vi "Get default digital audio protocol settings.vi"(11 "PCM Interfaces":T6) -> (3 "digital audio protocol settings":T1={"number of channels"=0, "data justification"=enum."Left Justified", "endianness"=enum."LSB First", "channel length"=0, "bit depth"=0, "frame clock rate"=0.0, "bit clock edge sync"=enum."Falling", "master clock rate"=0.0, "Logic Level"=enum."1.2 V", "frame sync edge for channel 0"=enum."Rising", "Channel 0 Offset"=0})   [LabVIEW 2021]
uses:
  Program Files/National Instruments/LabVIEW 2021/examples/Digital Audio Acquisition and Generation Toolkit/subVIs/PCM Interface Type.ctl
  digital audio protocol settings.ctl
  <vilib>/PDM Acquisition Toolkit/shared/controls/PCM Data Justification.ctl
  <vilib>/PDM Acquisition Toolkit/shared/controls/PCM Bit Endianness.ctl
  <vilib>/PDM Acquisition Toolkit/shared/controls/Digital Edge.ctl
  <vilib>/PDM Acquisition Toolkit/host/Classes/Session/Controls/Logic Levels.ctl
  <vilib>/PDM Acquisition Toolkit/shared/PDM Shared.lvlib
  <vilib>/PDM Acquisition Toolkit/host/Classes/Session/DecoderSession.lvclass
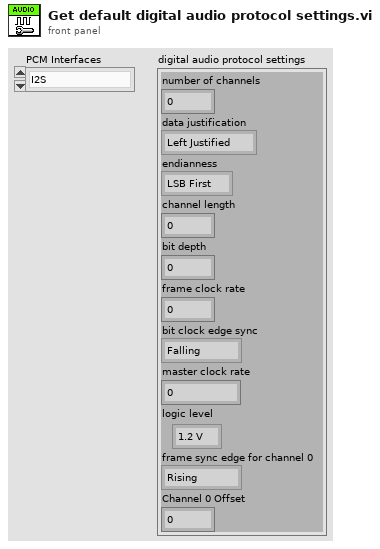
[diagram p1: front panel]
types:
  T1 = typedef "digital audio protocol settings.ctl" = cluster{"number of channels":u16, "data justification":T2, "endianness":T3, "channel length":u16, "bit depth":u8, "frame clock rate":dbl, "bit clock edge sync":T4, "master clock rate":dbl, "Logic Level":T5, "frame sync edge for channel 0":T4, "Channel 0 Offset":u16}
  T2 = typedef "PDM Shared.lvlib/PCM Data Justification.ctl" = enum16{"Left Justified", "Right Justified"}
  T3 = typedef "PDM Shared.lvlib/PCM Bit Endianness.ctl" = enum16{"MSB First", "LSB First"}
  T4 = typedef "PDM Shared.lvlib/Digital Edge.ctl" = enum8{"Rising", "Falling"}
  T5 = typedef "PDM Acquisition Class Library.lvlib/DecoderSession.lvclass/Logic Levels.ctl" = enum16{"3.3 V", "1.8 V", "1.2 V"}
  T6 = typedef "PCM Interface Type.ctl" = enum16{"I2S", "Left Justified", "Right Justified", "TDM 4 Channel", "TDM 6 Channel", "TDM 8 Channel", "DSP mode", "DSP mode with 1 bit delay", "PCM Short Frame", "PCM Long Frame"}
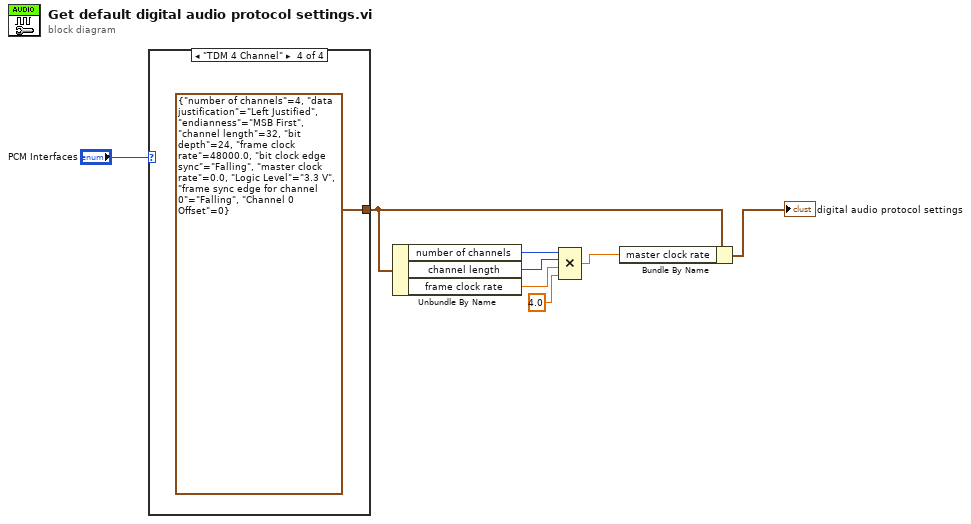
[diagram p0: block diagram]
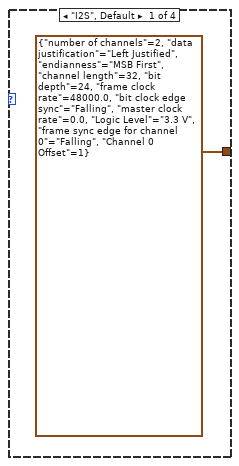
[diagram p2: hidden frame]
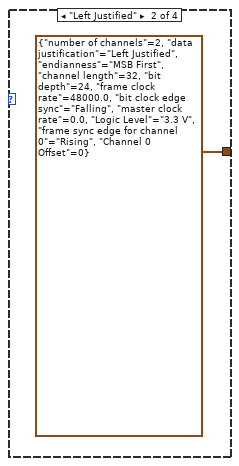
[diagram p3: hidden frame]
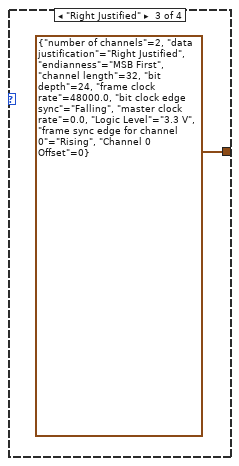
[diagram p4: hidden frame]
diagram:
  n1 = case shown="\"TDM 4 Channel\"" "PCM Interfaces" {
    tunnel: [T1 {"number of channels"=2, "data justification"=enum."Left Justified", "endianness"=enum."MSB First", "channel length"=32, "bit depth"=24, "frame clock rate"=48000.0, "bit clock edge sync"=enum."Falling", "master clock rate"=0.0, "Logic Level"=enum."3.3 V", "frame sync edge for channel 0"=enum."Falling", "Channel 0 Offset"=1} ("Cluster") T1 {"number of channels"=2, "data justification"=enum."Left Justified", "endianness"=enum."MSB First", "channel length"=32, "bit depth"=24, "frame clock rate"=48000.0, "bit clock edge sync"=enum."Falling", "master clock rate"=0.0, "Logic Level"=enum."3.3 V", "frame sync edge for channel 0"=enum."Rising", "Channel 0 Offset"=0} ("Cluster") T1 {"number of channels"=2, "data justification"=enum."Right Justified", "endianness"=enum."MSB First", "channel length"=32, "bit depth"=24, "frame clock rate"=48000.0, "bit clock edge sync"=enum."Falling", "master clock rate"=0.0, "Logic Level"=enum."3.3 V", "frame sync edge for channel 0"=enum."Rising", "Channel 0 Offset"=0} ("Cluster") T1 {"number of channels"=4, "data justification"=enum."Left Justified", "endianness"=enum."MSB First", "channel length"=32, "bit depth"=24, "frame clock rate"=48000.0, "bit clock edge sync"=enum."Falling", "master clock rate"=0.0, "Logic Level"=enum."3.3 V", "frame sync edge for channel 0"=enum."Falling", "Channel 0 Offset"=0} ("Cluster")] -> w7
    frame "I2S", Default {
    }
    frame "Left Justified" {
    }
    frame "Right Justified" {
    }
    frame "TDM 4 Channel" {
    }
  }
  n2 = Unbundle By Name(w7) -> ("number of channels"=w5:u16, "channel length"=w4:u16, "frame clock rate"=w3:dbl)
  n3 = Compound Arithmetic op=MULTIPLY(w5, w4, w3, 4.0 ("value")) -> (w1:dbl)
  n4 = Bundle By Name(cluster=w7, "master clock rate"=w1) -> (→"digital audio protocol settings":T1)
